vi "Scan For App Projects.vi"(8 "error in":errorcluster) -> (0 "error out":errorcluster)   [LabVIEW 2019, in "Panther Dashboard.lvlib"]
uses:
  Panther Dashboard.lvlib
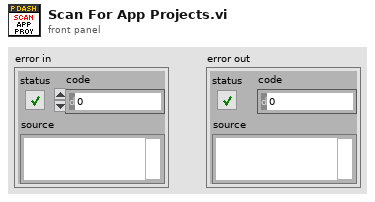
[diagram p1: front panel]
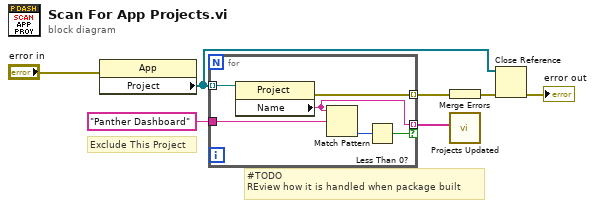
[diagram p0: block diagram]
diagram:
  # "#TODO\nREview how it is handled when package built"
  # "Exclude This Project"
  n1 = property class="App"(error in="error in") -> ("Project"=w4:refnum<vi>[])  [unwired: 1 in, 2 out]
  n2 = for {
    tunnel: w4 -> [w13] mode=indexing
    tunnel: [w12] -> w6 mode=indexing if=w9
    tunnel: "Panther Dashboard" -> [w11]
    tunnel: [w8] -> w2 mode=indexing
    n3 = property class="Project"(reference=w13) -> (error out=w8:errorcluster, "Name"=w12:string)  [unwired: 1 in, 1 out]
    n4 = Match Pattern(string=w12, regular expression=w11) -> (offset past match=w10:i32)  [unwired: 1 in, 3 out]
    n5 = Less Than 0?(x=w10) -> (x < 0?=w9:bool)
  }
  n6 = Merge Errors(w2) -> (w1:errorcluster)
  n7 = call "Projects Updated.vi"("Projects"=w6) -> ()  [unwired: 10 in, 1 out]
  n8 = Close Reference(reference=w4, error in (no error)=w1) -> (error out=→"error out":errorcluster)
